vi "Debug_SetSpeed.vi"(8 "error in (no error)":errorcluster, 10 "Speed":u32, 11 "SpinCoater in":refnum<class "SpinCoater.lvclass">) -> (0 "error out":errorcluster, 3 "SpinCoater out":refnum<class "SpinCoater.lvclass">)   [LabVIEW 2020, in "SpinCoater.lvclass"]
uses:
  <instrlib>/Classes/SpinCoater/SpinCoater.lvclass
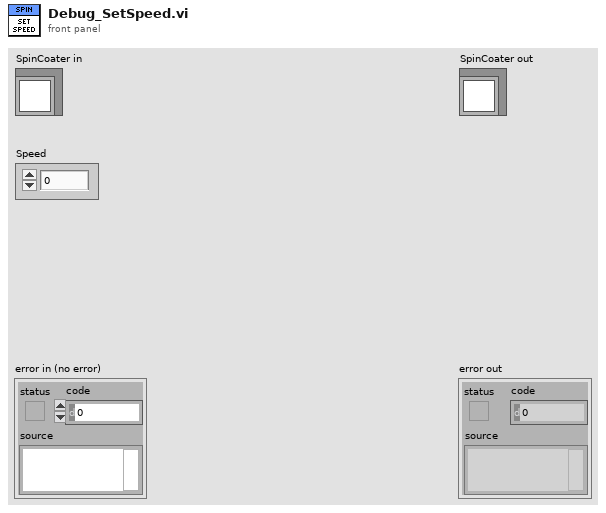
[diagram p1: front panel]
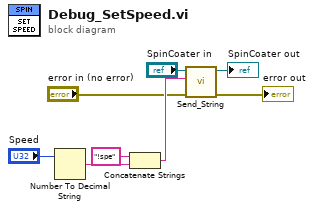
[diagram p0: block diagram]
diagram:
  n1 = Number To Decimal String(number="Speed") -> (decimal integer string=w8:string)  [unwired: 1 in]
  n2 = Concatenate Strings("!spe" ("string"), w8) -> (w4:string)
  n3 = call-dynamic "Send_String.vi"("error in (no error)"="error in (no error)", "String"=w4, "SpinCoater in"="SpinCoater in") -> ("error out"=→"error out":errorcluster, "SpinCoater out"=→"SpinCoater out":refnum<class "SpinCoater.lvclass">)  [unwired: 6 in, 1 out]
